vi "Audio Test.Generate Sine Sweep.vi"(8 "error in":errorcluster, 10 "Cal Data":path, 11 "Sine Sweep Params":T2={"Duration(s)"=2.0, "Amplitude"=1.0, "Freq Start"=20.0, "Freq End"=20000.0, "Samples/Sec"=44100.0} {"Amplitude" min=0.0 max=1.0 step=0.1}) -> (0 "error out":errorcluster, 1 "Sweep Attribues":T1, 2 "Play Duration":dbl, 3 "SweepWvfrm":waveform(dbl))   [LabVIEW 2018]
uses:
  TypeDefs/AudioTest.Config, Sine Sweep Params.ctl
  TypeDefs/AudioTest.Sweep Attributes.ctl
  <vilib>/addons/_NISVFA/_Generation/Signal Generation/SV Signal/SV Signal.lvclass/SV Signal.ctl
  <vilib>/addons/_NISVFA/_Generation/Signal Generation/SV Signal/Write Leading Synchronization Pulse Enable.vi
  <vilib>/addons/_NISVFA/_Generation/Signal Generation/SV Signal/Write Ramp-Up.vi
  <vilib>/addons/_NISVFA/_Generation/Signal Generation/SV Signal/Write Ramp-Down.vi
  <vilib>/addons/_NISVFA/_Generation/Signal Generation/SV Continuous Sweep/SV Continuous Sweep.lvclass
  C:/Program Files (x86)/National Instruments/LabVIEW 2018/vi.lib/addons/_NISVFA/_Generation/Signal Generation/SV Signal/SV Signal.lvclass
  <vilib>/addons/_NISVFA/_Generation/Signal Generation/SV Continuous Sweep/Configure Continuous Sweep.vi
  <vilib>/addons/_NISVFA/_Generation/Signal Generation/SV Signal/Write Ramp Parameters.vi
  <vilib>/addons/_NISVFA/_Generation/Signal Generation/SV Signal/Write DC Offset.vi
  <vilib>/addons/_NISVFA/_Generation/Signal Generation/SV Signal/Write Transition Profile.vi
  <vilib>/addons/_NISVFA/_Generation/Signal Generation/SV Signal/Write Pre-Measurement Settling Duration.vi
  <vilib>/addons/_NISVFA/_Generation/Signal Generation/SV Signal/Write Post-Measurement Settling Duration.vi
  <vilib>/addons/_NISVFA/_Generation/Signal Generation/SV Signal/Write Sample Rate.vi
  <vilib>/addons/_NISVFA/_Generation/Signal Generation/SV Signal/SV Signal.lvclass
panel:
  in  "Sample Rate (Hz)":dbl
  out "S/s":dbl
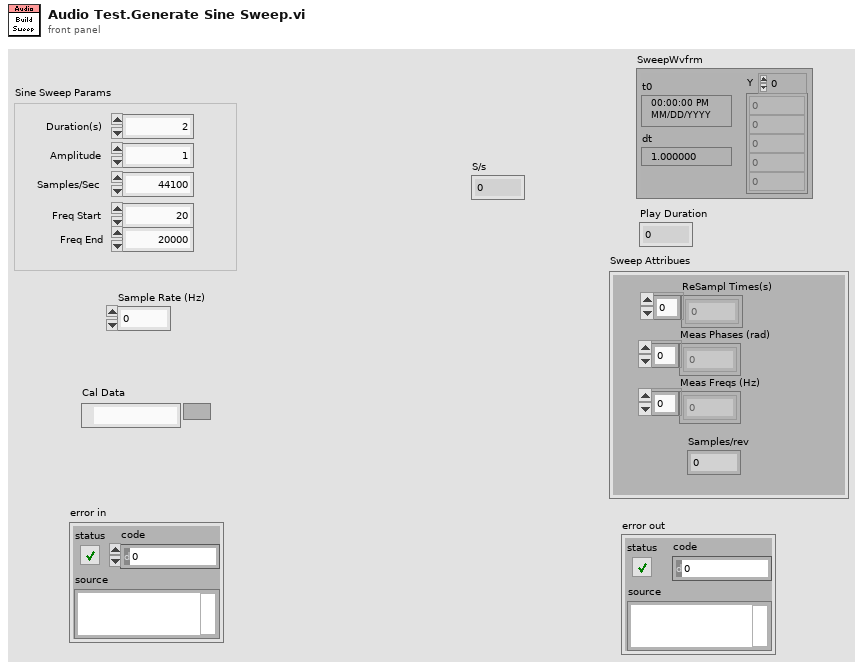
[diagram p1: front panel]
types:
  T1 = typedef "AudioTest.Sweep Attributes.ctl" = cluster{"ReSampl Times(s)":dbl[], "Meas Phases (rad)":dbl[], "Meas Freqs (Hz)":dbl[], "Samples/rev":i32}
  T2 = typedef "AudioTest.Config, Sine Sweep Params.ctl" = cluster{"Duration(s)":dbl, "Amplitude":dbl, "Freq Start":dbl, "Freq End":dbl, "Samples/Sec":dbl}
  T3 = cluster{"profile":enum16{"Linear", "Half cosine"}, "durations [s]":cluster{"ramp-up":dbl, "transition":dbl, "ramp-down":dbl}}
  T4 = cluster{"start frequency":dbl, "stop frequency":dbl, "number of steps":i32}
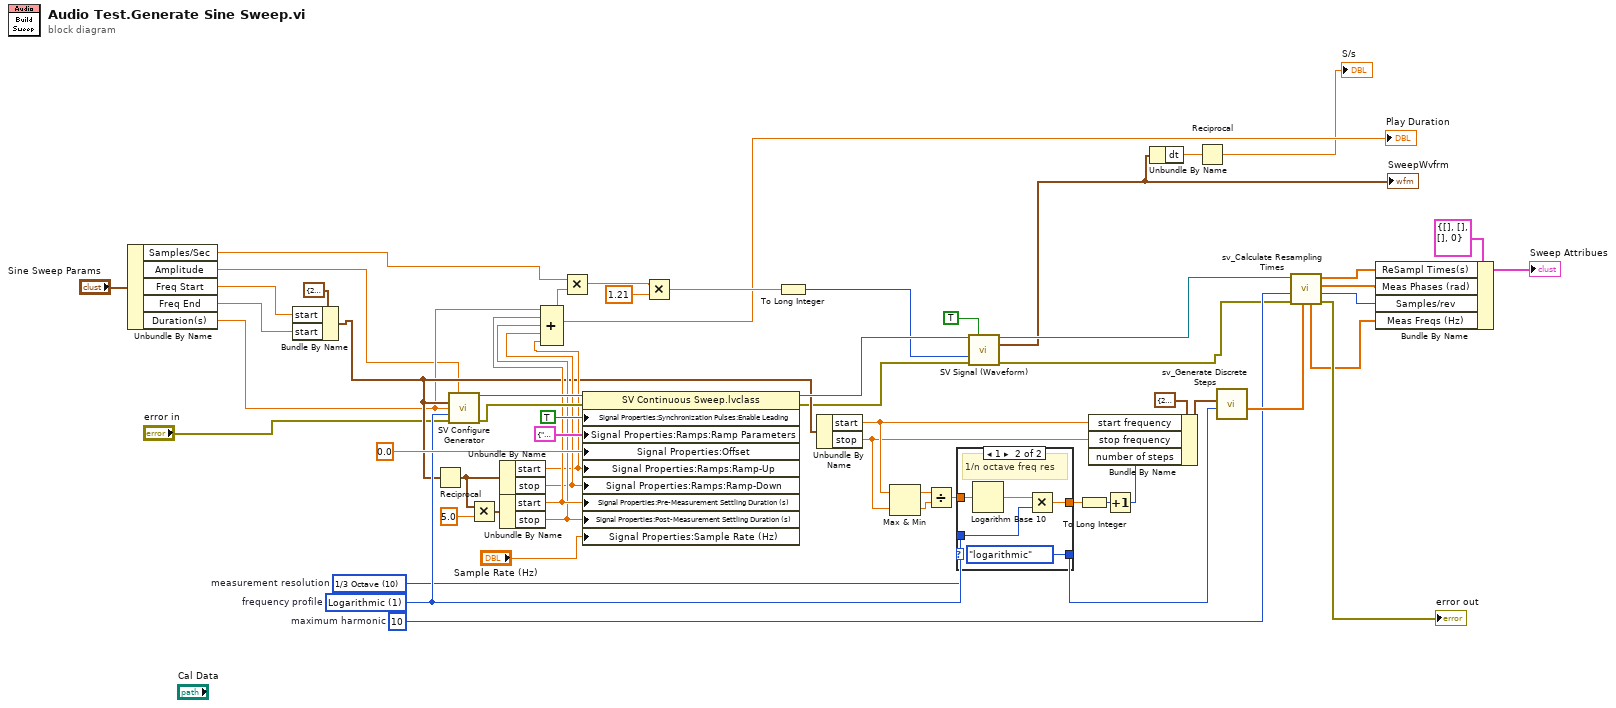
[diagram p0: block diagram]
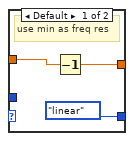
[diagram p2: hidden frame]
diagram:
  w35 = u16 10 items=["1/3 Octave"=10, "1/6 Octave"=20, "1/12 Octave"=40, "1/24 Octave"=80, "1/48 Octave"=160]  # measurement resolution
  w38 = u16 1 items=["Linear", "Logarithmic"]  # frequency profile
  w36 = 10  # maximum harmonic
  n1 = Unbundle By Name("Sine Sweep Params") -> ("Samples/Sec"=w20:dbl, "Amplitude"=w2:dbl, "Freq Start"=w17:dbl, "Freq End"=w16:dbl, "Duration(s)"=w14:dbl)
  n2 = Bundle By Name(cluster=cluster{"start":dbl, "stop":dbl} {"start"=20000.0, "stop"=40.0} ("frequency range"), "start"=w17, "start"=w16) -> (w15:cluster{"start":dbl, "stop":dbl})
  n3 = Reciprocal(x=w15) -> (1/x=w50:cluster{"start":dbl, "stop":dbl})
  n4 = call-poly <vilib>:"SV Configure Generator.vi"("amplitude"=w2, "frequency range [Hz]"=w15, "duration [s]"=w14, "profile"=w38, "error in (no error)"="error in") -> ("signal configuration"=w57:refnum<class "SV Continuous Sweep.lvclass">, "error out"=w55:errorcluster)  [unwired: 9 in]
  n5 = Multiply(x=w50, y=5.0 ("stop")) -> (x*y=w51:cluster{"start":dbl, "stop":dbl})
  n6 = Unbundle By Name(w50) -> ("start"=w26:dbl, "stop"=w27:dbl)
  n7 = Unbundle By Name(w51) -> ("start"=w30:dbl, "stop"=w29:dbl)
  n8 = Compound Arithmetic op=ADD(w14, w30, w29, w27, w26) -> (w22:dbl)
  "Play Duration" <- w22
  n9 = Multiply(x=w20, y=w22) -> (x*y=w25:dbl)
  n10 = property class="SV Continuous Sweep.lvclass"(reference=w57, error in=w55, "Signal Properties:Synchronization Pulses:Enable Leading"=TRUE ("Synchronization Pulses:Enable Leading"), "Signal Properties:Ramps:Ramp Parameters"=T3 {"profile"=enum."Half cosine", "durations [s]"={"ramp-up"=0.01, "transition"=0.0, "ramp-down"=0.01}} ("Ramp Parameters"), "Signal Properties:Offset"=0.0 ("DC offset"), "Signal Properties:Ramps:Ramp-Up"=w26, "Signal Properties:Ramps:Ramp-Down"=w27, "Signal Properties:Pre-Measurement Settling Duration (s)"=w30, "Signal Properties:Post-Measurement Settling Duration (s)"=w29, "Signal Properties:Sample Rate (Hz)"="Sample Rate (Hz)") -> (reference out=w34:refnum<class "SV Continuous Sweep.lvclass">, error out=w7:errorcluster)
  n11 = Multiply(x=w25, y=1.21) -> (x*y=w23:dbl)
  n12 = To Long Integer(number=w23) -> (32bit integer=w28:i32)
  n13 = Unbundle By Name(w15) -> ("start"=w42:dbl, "stop"=w41:dbl)
  n14 = Max & Min(x=w42, y=w41) -> (max(x,y)=w47:dbl, min(x,y)=w46:dbl)
  n15 = Divide(x=w47, y=w46) -> (x/y=w45:dbl)
  n16 = case shown="1" w38 {
    tunnel: w45 -> [w59 w65]
    tunnel: [w58 w63] -> w44
    tunnel: [enum16{"linear", "logarithmic"}."linear" ("spacing") enum16{"linear", "logarithmic"}."logarithmic" ("spacing")] -> w39
    tunnel: w35 -> [_ w61]
    frame Default {
      # "use min as freq res"
      n17 = Decrement(x=w59) -> (x-1=w58:dbl)
    }
    frame 1 {
      # "1/n octave freq res"
      n18 = Logarithm Base 10(1:w65) -> (0:w64:dbl)
      n19 = Multiply(x=w64, y=w61) -> (x*y=w63:dbl)
    }
  }
  n20 = call-dynamic "SV Signal (Waveform).vi"("signal configuration"=w34, "reset"=TRUE, "samples"=w28, "error in (no error)"=w7) -> ("signal configuration"=w32:refnum<class "SV Continuous Sweep.lvclass">, "output waveform"=w5:waveform(dbl), "error out"=w31:errorcluster)  [unwired: 6 in, 3 out]
  "SweepWvfrm" <- w5
  n21 = To Long Integer(number=w44) -> (32bit integer=w43:i32)
  n22 = Increment(x=w43) -> (x+1=w40:i32)
  n23 = Bundle By Name(cluster=T4 {"start frequency"=20.0, "stop frequency"=20000.0, "number of steps"=100} ("sweep frequencies"), "start frequency"=w42, "stop frequency"=w41, "number of steps"=w40) -> (w48:T4)
  n24 = Unbundle By Name(w5) -> ("dt"=w4:dbl)
  n25 = Reciprocal(x=w4) -> (1/x=→"S/s":dbl)
  n26 = call <vilib>:"sv_Generate Discrete Steps.vi"("spacing"=w39, "steps"=w48) -> ("frequency list"=w37:dbl[])  [unwired: 8 in, 1 out]
  n27 = call "sv_Calculate Resampling Times.vi"("measurement frequencies in (Hz)"=w37, "error in"=w31, "maximum harmonic"=w36, "continuous sweep configuration"=w32) -> ("error out"=→"error out":errorcluster, "samples/rev"=w9:i32, "measurement phases (rad)"=w10:dbl[], "resampling times (s)"=w11:dbl[], "measurement frequencies (Hz)"=w8:dbl[])  [unwired: 1 in, 2 out]
  n28 = Bundle By Name(cluster=T1 {"ReSampl Times(s)"=[], "Meas Phases (rad)"=[], "Meas Freqs (Hz)"=[], "Samples/rev"=0} ("Sweep Attribues"), "ReSampl Times(s)"=w11, "Meas Phases (rad)"=w10, "Samples/rev"=w9, "Meas Freqs (Hz)"=w8) -> (→"Sweep Attribues":T1)
